vi "InitImages.vi"(11 "camera id":string) -> (1 "test panel image":T1, 2 "scaled image":T1, 3 "raw image":T1)   [LabVIEW 2017, in "IrAcquisition.lvlib"]
uses:
  <vilib>/addons/InsightCM/Devices/Shared/Ir/IrAcquisition/IrAcquisition.lvlib
  <vilib>/vision/Image Controls.llb/IMAQ Image.ctl
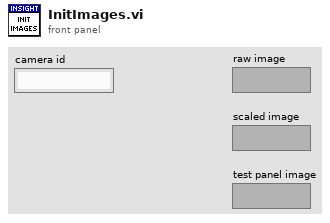
[diagram p1: front panel]
types:
  T1 = typedef "IMAQ Image.ctl" = refnum<image>
  T2 = typedef "Image Type" = u32
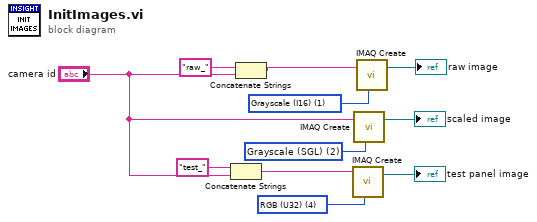
[diagram p0: block diagram]
diagram:
  w5 = T2 4 items=["Grayscale (U8)", "Grayscale (I16)", "Grayscale (SGL)", "Complex (CSG)", "RGB (U32)", "HSL (U32)", "RGB (U64)", "Grayscale (U16)"] ("Image Type")
  w3 = T2 2 items=["Grayscale (U8)", "Grayscale (I16)", "Grayscale (SGL)", "Complex (CSG)", "RGB (U32)", "HSL (U32)", "RGB (U64)", "Grayscale (U16)"] ("Image Type")
  w2 = T2 1 items=["Grayscale (U8)", "Grayscale (I16)", "Grayscale (SGL)", "Complex (CSG)", "RGB (U32)", "HSL (U32)", "RGB (U64)", "Grayscale (U16)"] ("Image Type")
  n1 = Concatenate Strings("test_" ("initial string"), "camera id") -> (w10:string)
  n2 = Concatenate Strings("raw_" ("initial string"), "camera id") -> (w8:string)
  n3 = call "IMAQ Create"("Image Name"=w10, "Image Type"=w5) -> ("New Image"=→"test panel image":T1)  [unwired: 2 in, 2 out]
  n4 = call "IMAQ Create"("Image Name"="camera id", "Image Type"=w3) -> ("New Image"=→"scaled image":T1)  [unwired: 2 in, 2 out]
  n5 = call "IMAQ Create"("Image Name"=w8, "Image Type"=w2) -> ("New Image"=→"raw image":T1)  [unwired: 2 in, 2 out]
